vi "check_cancellation_on.vi"(6 "Reset":bool, 11 "Mode controls in":T1) -> (3 "Mode controls out":T1)   [LabVIEW 2012]
uses:
  mode_conrols.ctl
  <vilib>/Analysis/Matrix/Numeric/Conversions/Array To Matrix - RA2.vi
  utilities/labview/magnitude_dbl.vi
  <vilib>/Analysis/Matrix/NI_Matrix.lvlib
panel:
  in  "Delay length":i32=3
  in  "Velocity cutoff (mm/sec)":sgl=10.0
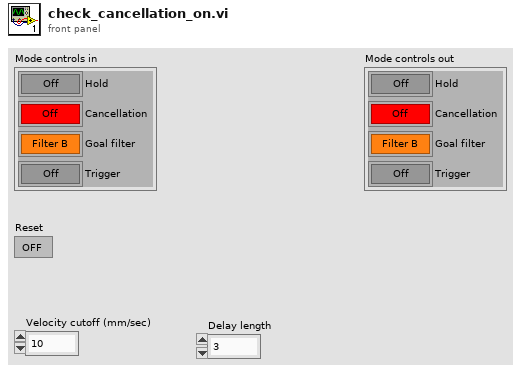
[diagram p1: front panel]
types:
  T1 = typedef "mode_conrols.ctl" = cluster{"Hold":bool, "Cancellation":bool, "Goal filter":bool, "Trigger":bool}
  T2 = typedef "NI_Matrix.lvlib/RealMatrix.ctl" = dbl[][]
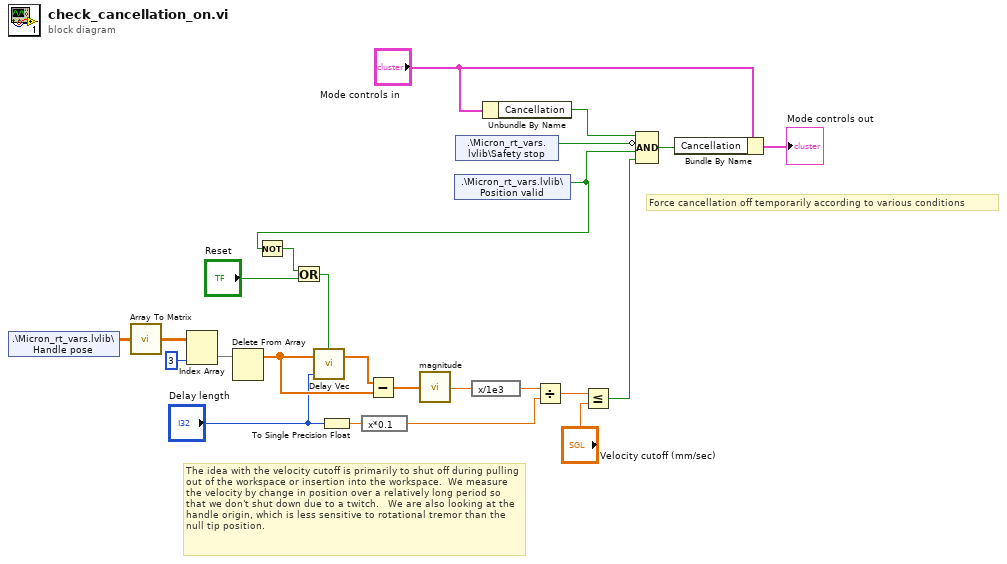
[diagram p0: block diagram]
diagram:
  # "The idea with the velocity cutoff is primarily to shut off during pulling out of the workspace or insertion into the workspace.  We measure the velocity by change in position over a relatively long period so that we don't shut down due to a twitch.   We are also looking at the handle origin, which is less sensitive to rotational tremor than the null tip position."
  # "Force cancellation off temporarily according to various conditions"
  n1 = shared-variable ".\\Micron_rt_vars.lvlib\\Handle pose"() -> (w19:sgl[][])  [unwired: 2 out]
  n2 = call-poly <vilib>:"Array To Matrix.vi"("Real 2D Array"=w19) -> ("Real Matrix"=w18:T2)
  n3 = Index Array(array=w18, index (col)=3 ("disabled index (col)")) -> (element=w16:dbl[])  [unwired: 1 in]
  n4 = Delete From Array(array=w16) -> (array with subset deleted=w14:dbl[])  [unwired: 2 in, 1 out]
  n5 = To Single Precision Float(number="Delay length") -> (single precision float=w2:sgl)
  n6 = expression code="x*0.1"(w2) -> (w10:sgl)
  n7 = shared-variable ".\\Micron_rt_vars.lvlib\\Position valid"() -> (w1:bool)  [unwired: 2 out]
  n8 = Not(x=w1) -> (.not. x?=w4:bool)
  n9 = Or(x=w4, y="Reset") -> (x .or. y?=w5:bool)
  n10 = call "Delay Vec.vi"("initialize"=w5, "Delay length"="Delay length", "X"=w14) -> ("Delayed X"=w15:sgl[])  [unwired: 2 in]
  n11 = Subtract(x=w15, y=w14) -> (x-y=w13:dbl[])
  n12 = call-poly "magnitude.vi"("vector"=w13) -> ("vector magnitude"=w12:dbl)  [unwired: 4 in]
  n13 = shared-variable ".\\Micron_rt_vars.lvlib\\Safety stop"() -> (w20:bool)  [unwired: 2 out]
  n14 = expression code="x/1e3"(w12) -> (w11:dbl)
  n15 = Unbundle By Name("Mode controls in") -> ("Cancellation"=w22:bool)
  n16 = Divide(x=w11, y=w10) -> (x/y=w9:dbl)
  n17 = Less Or Equal?(x=w9, y="Velocity cutoff (mm/sec)") -> (x <= y?=w7:bool)
  n18 = Compound Arithmetic op=AND(w22, invert w20, w1, w7) -> (w21:bool)
  n19 = Bundle By Name(cluster="Mode controls in", "Cancellation"=w21) -> (→"Mode controls out":T1)
